vi "Write Data Test.vi"(8 "error in (no error)":errorcluster caption="entrée d'erreur (pas d'erreur)", 11 "Database Altyor en entrée":refnum<class "Database Altyor.lvclass">) -> (0 "error out":errorcluster caption="sortie d'erreur", 3 "Database Altyor en sortie":refnum<class "Database Altyor.lvclass">)   [LabVIEW 2020, in "Library Instrument & Equipement.lvlib" / "Library Database.lvlib" / "Database Altyor.lvclass"]
uses:
  Database Altyor.lvclass
  C:/Users/ngarcin/OneDrive - Altyor/Standard TB/Suite TB45/Class/Database/Database drivers/Database Drivers.lvclass
  Commun VI/TypeDef/Variable Printable.ctl
  Commun VI/Library Commun.lvlib
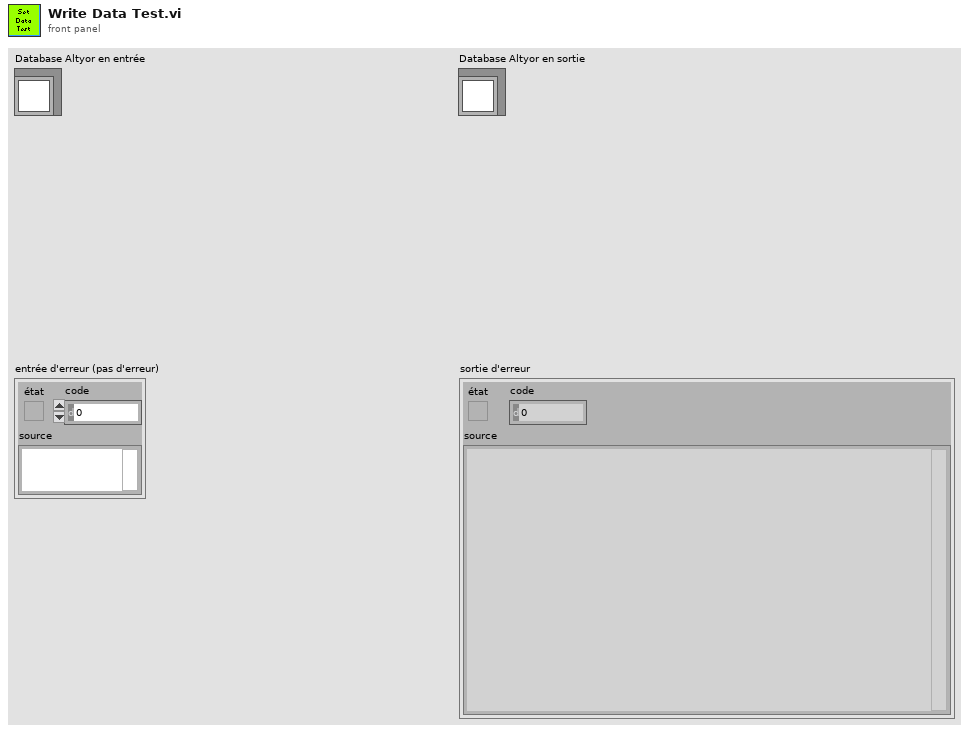
[diagram p1: front panel]
types:
  T1 = typedef "Variable Printable.ctl" = string
  T2 = enum16{"Get Variable", "Get All Variables", "Set Variable", "Delete Variable", "Delete All Variable"}
  T3 = cluster{"Key_Test":u32, "idTest":u32, "MainTest":string, "Name":string, "StartOfTest":string, "EndOfTest":string, "Result":string, "LimitMax":string, "Value":string, "LimitMin":string, "Type":string}
  T4 = cluster{"Key_Test":u32, "idTest":u32, "MainTest":string, "Name":string, "StartOfTest":string, "EndOfTest":string, "Result":string, "LimitMax":string, "Value":string, "LimitMin":string, "Type":string}[]
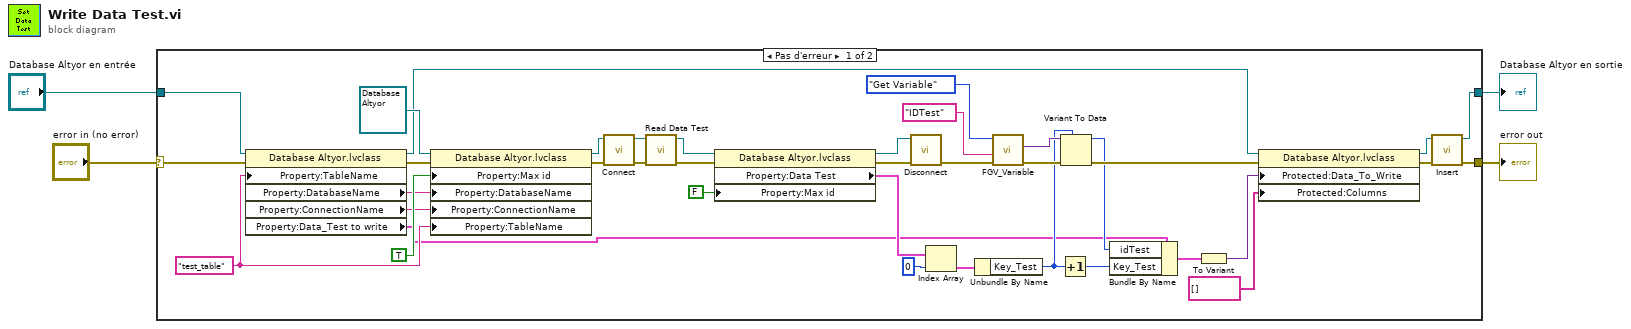
[diagram p0: block diagram]
diagram:
  n1 = case shown="Pas d'erreur" "error in (no error)" {
    selector: "error in (no error)" -> [w37 w44]
    tunnel: [w39 w44] -> w2
    tunnel: [w40 w43] -> w1
    tunnel: "Database Altyor en entrée" -> [w38 w43]
    frame No Error {
      w6 = "test_table" ("TableName")
      n2 = property class="Database Altyor.lvclass"(reference=w38, error in=w37, "Property:TableName"=w6) -> (reference out=w10:refnum<class "Database Altyor.lvclass">, error out=w35:errorcluster, "Property:DatabaseName"=w7:string, "Property:ConnectionName"=w8:string, "Property:Data_Test to write"=w5:T3)
      n3 = property class="Database Altyor.lvclass"(reference=refnum<class "Database Altyor.lvclass"> refnum ("Library Database.lvlib:Database Altyor.lvclass"), error in=w35, "Property:Max id"=TRUE ("Max id"), "Property:DatabaseName"=w7, "Property:ConnectionName"=w8, "Property:TableName"=w6) -> (reference out=w16:refnum<class "Database Altyor.lvclass">, error out=w13:errorcluster)
      n4 = call-dynamic "Connect.vi"("error in (no error)"=w13, "Database Altyor en entrée"=w16) -> ("error out"=w14:errorcluster, "Database Altyor en sortie"=w15:refnum<class "Database Altyor.lvclass">)  [unwired: 8 in]
      n5 = call-dynamic "Read Data Test.vi"("error in (no error)"=w14, "Database Altyor en entrée"=w15) -> ("error out"=w20:errorcluster, "Database Altyor en sortie"=w19:refnum<class "Database Altyor.lvclass">)  [unwired: 8 in]
      n6 = property class="Database Altyor.lvclass"(reference=w19, error in=w20, "Property:Max id"=FALSE ("Max id")) -> (reference out=w12:refnum<class "Database Altyor.lvclass">, error out=w11:errorcluster, "Property:Data Test"=w31:T4)
      n7 = call-dynamic "Disconnect.vi"("error in (no error)"=w11, "Database Altyor en entrée"=w12) -> ("error out"=w9:errorcluster)  [unwired: 8 in, 1 out]
      n8 = Index Array(array=w31, index=0 ("indice")) -> (element=w34:T3)
      n9 = Unbundle By Name(w34) -> ("Key_Test"=w23:u32)
      n10 = call "FGV_Variable.vi"("error in (no error)"=w9, "Variable"=T1 "IDTest", "Function"=T2."Get Variable") -> ("error out"=w27:errorcluster, "Data Out"=w24:variant)  [unwired: 6 in, 1 out]
      n11 = Increment(x=w23) -> (x+1=w28:u32)
      n12 = Variant To Data(error in=w27, type=w23, Variant=w24) -> (data=w22:u32, error out=w25:errorcluster)
      n13 = Bundle By Name(cluster=w5, "idTest"=w22, "Key_Test"=w28) -> (w32:T3)
      n14 = To Variant(anything=w32) -> (Variant=w36:variant)
      n15 = property class="Database Altyor.lvclass"(reference=w10, error in=w25, "Protected:Data_To_Write"=w36, "Protected:Columns"=string[] [] ("Columns")) -> (reference out=w42:refnum<class "Database Altyor.lvclass">, error out=w41:errorcluster)
      n16 = call-dynamic "Insert.vi"("error in (no error)"=w41, "Database Drivers en entrée"=w42) -> ("error out"=w39:errorcluster, "Database Drivers en sortie"=w40:refnum<class "Database Altyor.lvclass">)  [unwired: 8 in]
    }
    frame Error {
    }
  }
  "error out" <- w2
  "Database Altyor en sortie" <- w1
